vi "rx_demo.vi"() -> ()   [LabVIEW 2023]
uses:
  <instrlib>/niUSRP/niUSRP Fetch Rx Data (CDB WDT).vi
panel:
  out "Waveform Graph":dbl[](graph)
  in  "stop":bool
  in  "number of samples":i64=100000
  in  "active antenna":string
  in  "gain":dbl format="%#_6f"
  in  "carrier frequency":dbl=100000.0 format="%#_6p"
  in  "IQ rate":dbl=100000.0 format="%#_6p"
  in  "device names":refnum<k15>
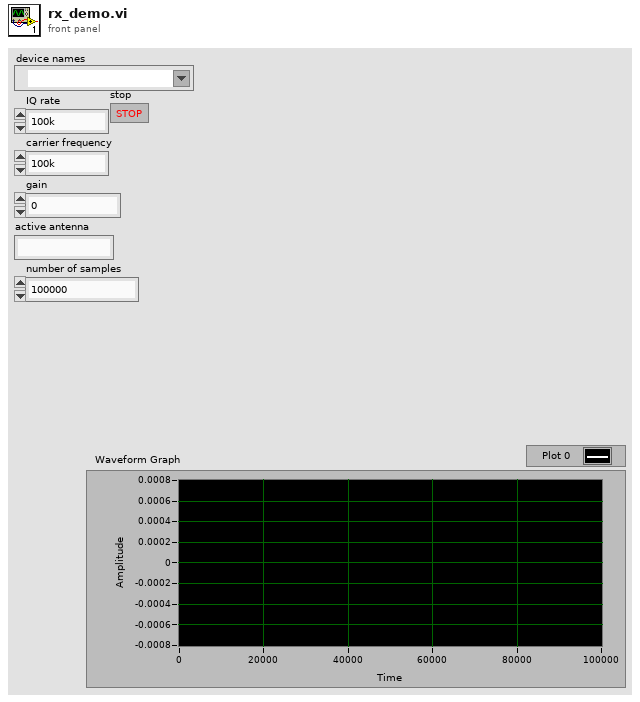
[diagram p1: front panel]
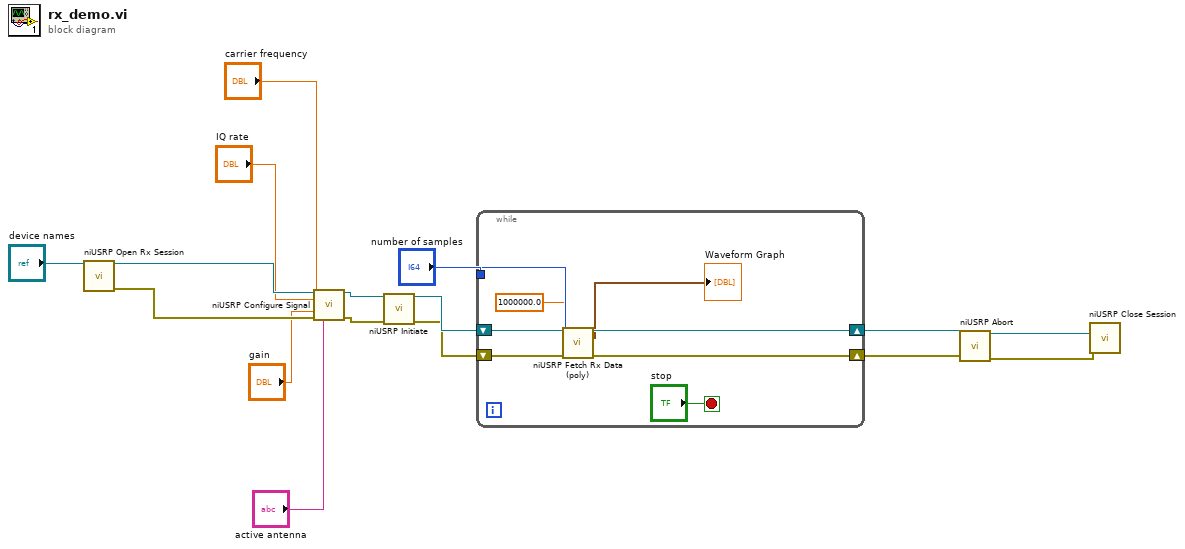
[diagram p0: block diagram]
diagram:
  n1 = call <instrlib>:"niUSRP Open Rx Session.vi"("device names"="device names") -> ("session handle out"=w8:refnum<k15>, "error out"=w7:errorcluster)  [unwired: 13 in]
  n2 = call <instrlib>:"niUSRP Configure Signal.vi"("session handle"=w8, "IQ rate"="IQ rate", "carrier frequency"="carrier frequency", "gain"="gain", "error in (no error)"=w7, "active antenna"="active antenna") -> ("session handle out"=w16:refnum<k15>, "error out"=w15:errorcluster)  [unwired: 5 in, 3 out]
  n3 = call <instrlib>:"niUSRP Initiate.vi"("session handle"=w16, "error in (no error)"=w15) -> ("session handle out"=w10:refnum<k15>, "error out"=w9:errorcluster)  [unwired: 12 in]
  n4 = while {
    tunnel: "number of samples" -> [w20]
    shift-right: [w24] -> w14
    shift-left: w10 -> [w22]
    shift-right: [w23] -> w13
    shift-left: w9 -> [w21]
    stop <- "stop" stop-if-true
    n5 = call-poly <instrlib>:"niUSRP Fetch Rx Data (poly).vi"("session handle"=w22, "number of samples"=w20, "timeout"=1000000.0, "error in (no error)"=w21) -> ("session handle out"=w24:refnum<k15>, "data"=→"Waveform Graph":waveform(cdb), "error out"=w23:errorcluster)  [unwired: 8 in, 1 out]
  }
  n6 = call <instrlib>:"niUSRP Abort.vi"("session handle"=w14, "error in (no error)"=w13) -> ("session handle out"=w12:refnum<k15>, "error out"=w11:errorcluster)  [unwired: 12 in]
  n7 = call <instrlib>:"niUSRP Close Session.vi"("session handle"=w12, "error in (no error)"=w11) -> ()  [unwired: 13 in, 1 out]
